vi "VI State.vi"(8 "error in (no error)":errorcluster, 11 "VI in":refnum<vi>) -> (0 "error out":errorcluster)   [LabVIEW 2015]
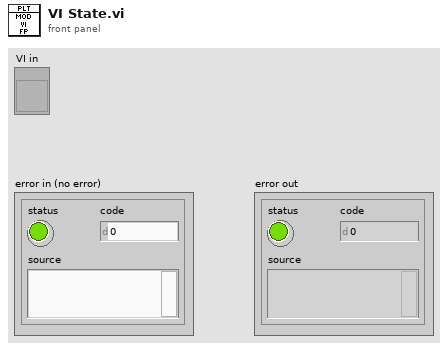
[diagram p1: front panel]
types:
  T1 = enum32{"invalid app kind", "Development System", "Run Time System", "Student Edition", "Embedded LabVIEW", "Evaluation", "Custom"}
  T2 = enum32{"Invalid", "Default", "Floating", "Floating/Auto-Hide", "Modal"}
  T3 = enum32{"Invalid", "Standard", "Closed", "Hidden", "Minimized", "Maximized"}
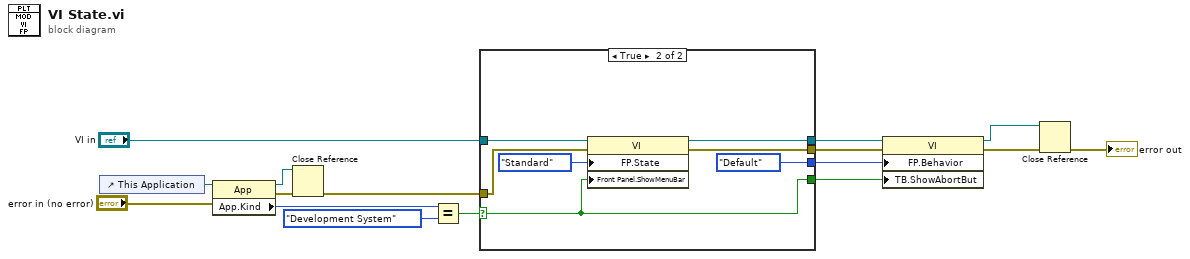
[diagram p0: block diagram]
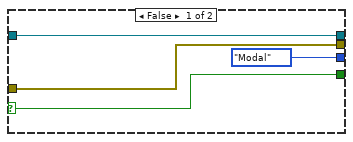
[diagram p2: hidden frame]
diagram:
  n1 = control-ref of="This Application"() -> (w15:refnum<vi>)
  n2 = property class="App"(reference=w15, error in="error in (no error)") -> (reference out=w5:refnum<vi>, error out=w16:errorcluster, "App.Kind"=w14:T1)
  n3 = Close Reference(reference=w5, error in (no error)=w16) -> (error out=w8:errorcluster)
  n4 = Equal?(x=w14, y=T1."Development System") -> (x = y?=w12:bool)
  n5 = case shown="True" w12 {
    selector: w12 -> [w18 w21]
    tunnel: "VI in" -> [w20 w26]
    tunnel: [w20 w22] -> w10
    tunnel: [T2."Modal" ("Front Panel Window:Behavior") T2."Default" ("Front Panel Window:Behavior")] -> w9
    tunnel: [w18 w21] -> w4
    tunnel: w8 -> [w17 w25]
    tunnel: [w17 w23] -> w7
    frame False {
    }
    frame True {
      n6 = property class="VI"(reference=w26, error in=w25, "FP.State"=T3."Standard" ("Front Panel Window:State"), "Front Panel.ShowMenuBar"=w21) -> (reference out=w22:refnum<vi>, error out=w23:errorcluster)
    }
  }
  n7 = property class="VI"(reference=w10, error in=w7, "FP.Behavior"=w9, "TB.ShowAbortBut"=w4) -> (reference out=w1:refnum<vi>, error out=w3:errorcluster)
  n8 = Close Reference(reference=w1, error in (no error)=w3) -> (error out=→"error out":errorcluster)
